vi "PIController.vi"(0 "Kp":dbl, 5 "Ti":dbl, 7 "setP":dbl, 9 "temp":dbl) -> (4 "Control Signal":dbl)   [LabVIEW 2019]
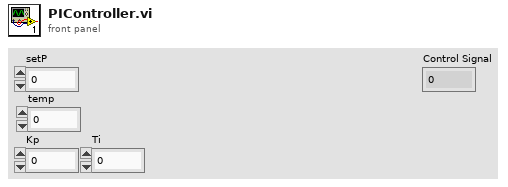
[diagram p1: front panel]
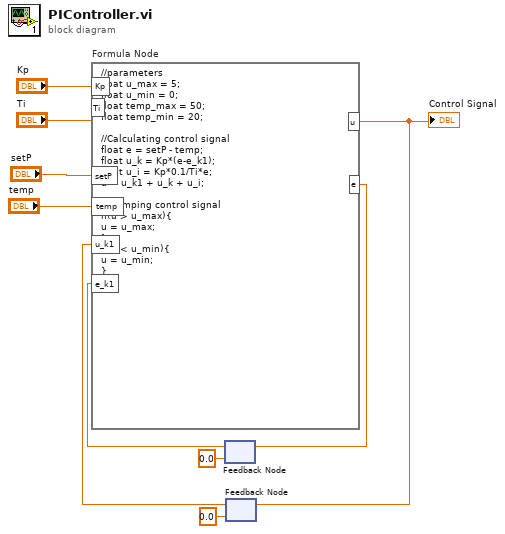
[diagram p0: block diagram]
diagram:
  n1 = feedback #1(0.0) -> (w5:dbl)
  n2 = feedback #2(0.0 ("u")) -> (w3:dbl)
  n3 = formula code="//parameters\nfloat u_max = 5;\nfloat u_min = 0;\nfloat temp_max = 50;\nfloat temp_min = 20;\n\n//Calculating control signal\nfloat e = setP - temp;\nfloat u_k = Kp*(e-e_k1);\nfloat u_i = Kp*0.1/Ti*e;\nu = u_k1 + u_k + u_i;\n\n//Clamping control signal\nif(u > u_max){\nu = u_max;\n}\nif(u < u_min){\nu = u_min;\n}"("setP"="setP", "temp"="temp", "u_k1"=w3, "Kp"="Kp", "Ti"="Ti", "e_k1"=w5) -> ("u"=w4:dbl, "e"=w6:dbl)
  "Control Signal" <- w4
  n4 = feedback-in #1(w6) -> ()
  n5 = feedback-in #2(w4) -> ()
